vi "FocalChecker.vi"() -> ()   [LabVIEW 2016]
panel:
  out "Spectrum mean normalized 5":dbl[](graph)
  in  "File Path 5":path
  out "Spectrum mean normalized 4":dbl[](graph)
  in  "File Path 4":path
  out "Spectrum mean normalized 3":dbl[](graph)
  in  "File Path 3":path
  out "Spectrum mean normalized 2":dbl[](graph)
  in  "File Path 2":path
  in  "length Y":i32
  in  "index Y":i32
  in  "length X":i32
  in  "index X":i32
  in  "Multiplicator":dbl
  out "Spectrum mean normalized":dbl[](graph)
  in  "File Path":path
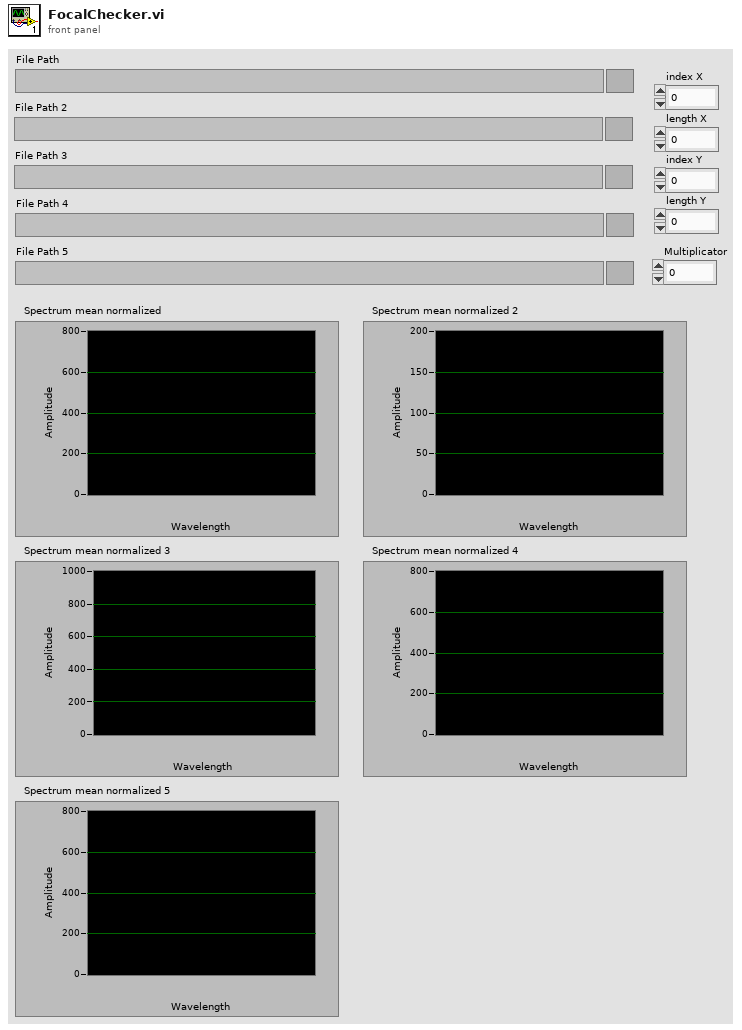
[diagram p1: front panel]
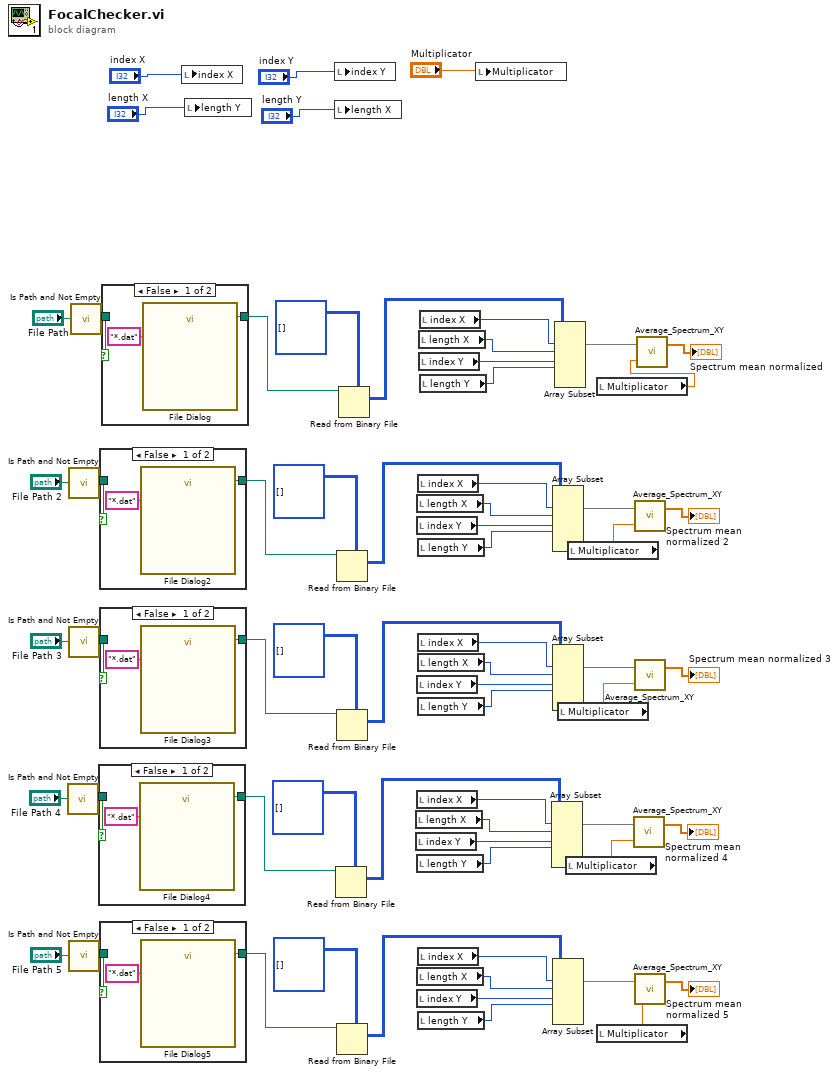
[diagram p0: block diagram]
diagram:
  n1 = call <vilib>:"Is Path and Not Empty.vi"("path"="File Path 4") -> ("Is Path and Not Empty?"=w26:bool)  [unwired: 4 in]
  n2 = call <vilib>:"Is Path and Not Empty.vi"("path"="File Path 2") -> ("Is Path and Not Empty?"=w48:bool)  [unwired: 4 in]
  n3 = call <vilib>:"Is Path and Not Empty.vi"("path"="File Path 3") -> ("Is Path and Not Empty?"=w37:bool)  [unwired: 4 in]
  n4 = call <vilib>:"Is Path and Not Empty.vi"("path"="File Path 5") -> ("Is Path and Not Empty?"=w15:bool)  [unwired: 4 in]
  n5 = call <vilib>:"Is Path and Not Empty.vi"("path"="File Path") -> ("Is Path and Not Empty?"=w64:bool)  [unwired: 4 in]
  n6 = case shown="False" w26 {
    tunnel: [w67 w68] -> w27
    tunnel: "File Path 4" -> [_ w68]
    frame False {
      n7 = call "File Dialog4"("pattern (all files)"="*.dat") -> ("selected path"=w67:path)  [unwired: 11 in, 3 out]
    }
    frame True {
    }
  }
  n8 = case shown="False" w48 {
    tunnel: [w70 w71] -> w49
    tunnel: "File Path 2" -> [_ w71]
    frame False {
      n9 = call "File Dialog2"("pattern (all files)"="*.dat") -> ("selected path"=w70:path)  [unwired: 11 in, 3 out]
    }
    frame True {
    }
  }
  n10 = case shown="False" w37 {
    tunnel: [w73 w74] -> w38
    tunnel: "File Path 3" -> [_ w74]
    frame False {
      n11 = call "File Dialog3"("pattern (all files)"="*.dat") -> ("selected path"=w73:path)  [unwired: 11 in, 3 out]
    }
    frame True {
    }
  }
  n12 = case shown="False" w15 {
    tunnel: [w76 w77] -> w16
    tunnel: "File Path 5" -> [_ w77]
    frame False {
      n13 = call "File Dialog5"("pattern (all files)"="*.dat") -> ("selected path"=w76:path)  [unwired: 11 in, 3 out]
    }
    frame True {
    }
  }
  n14 = case shown="False" w64 {
    tunnel: [w79 w80] -> w65
    tunnel: "File Path" -> [_ w80]
    frame False {
      n15 = call "File Dialog"("pattern (all files)"="*.dat") -> ("selected path"=w79:path)  [unwired: 11 in, 3 out]
    }
    frame True {
    }
  }
  n16 = local write "index X"("index X") -> ()
  n17 = local write "length Y"("length X") -> ()
  n18 = local write "index Y"("index Y") -> ()
  n19 = local write "length X"("length Y") -> ()
  n20 = Read from Binary File(5:u32[][][] [], 11:w27) -> (2:w21:u32[][][])  [unwired: 4 in, 3 out]
  n21 = Read from Binary File(5:u32[][][] [], 11:w49) -> (2:w43:u32[][][])  [unwired: 4 in, 3 out]
  n22 = Read from Binary File(5:u32[][][] [], 11:w38) -> (2:w32:u32[][][])  [unwired: 4 in, 3 out]
  n23 = Read from Binary File(5:u32[][][] [], 11:w16) -> (2:w10:u32[][][])  [unwired: 4 in, 3 out]
  n24 = Read from Binary File(5:u32[][][] [], 11:w65) -> (2:w59:u32[][][])  [unwired: 4 in, 3 out]
  n25 = local read "length X"() -> (w19:i32)
  n26 = local read "index Y"() -> (w18:i32)
  n27 = local read "length X"() -> (w41:i32)
  n28 = local read "index Y"() -> (w40:i32)
  n29 = local read "index Y"() -> (w29:i32)
  n30 = local read "index X"() -> (w20:i32)
  n31 = local read "length Y"() -> (w17:i32)
  n32 = local read "length X"() -> (w8:i32)
  n33 = local read "index Y"() -> (w7:i32)
  n34 = local read "index X"() -> (w42:i32)
  n35 = local read "length Y"() -> (w39:i32)
  n36 = local read "index X"() -> (w31:i32)
  n37 = local read "length X"() -> (w30:i32)
  n38 = local read "length Y"() -> (w28:i32)
  n39 = local read "index X"() -> (w9:i32)
  n40 = local read "length Y"() -> (w6:i32)
  n41 = local read "length X"() -> (w52:i32)
  n42 = local read "index Y"() -> (w51:i32)
  n43 = local read "index X"() -> (w53:i32)
  n44 = local read "length Y"() -> (w50:i32)
  n45 = local write "Multiplicator"("Multiplicator") -> ()
  n46 = Array Subset(array=w21, index (dim 0)=w20, length (dim 0)=w19, index (dim 1)=w18, length (dim 1)=w17) -> (w24:u32[][][])  [unwired: 2 in]
  n47 = Array Subset(array=w43, index (dim 0)=w42, length (dim 0)=w41, index (dim 1)=w40, length (dim 1)=w39) -> (w46:u32[][][])  [unwired: 2 in]
  n48 = Array Subset(array=w32, index (dim 0)=w31, length (dim 0)=w30, index (dim 1)=w29, length (dim 1)=w28) -> (w35:u32[][][])  [unwired: 2 in]
  n49 = Array Subset(array=w10, index (dim 0)=w9, length (dim 0)=w8, index (dim 1)=w7, length (dim 1)=w6) -> (w13:u32[][][])  [unwired: 2 in]
  n50 = Array Subset(array=w59, index (dim 0)=w53, length (dim 0)=w52, index (dim 1)=w51, length (dim 1)=w50) -> (w62:u32[][][])  [unwired: 2 in]
  n51 = local read "Multiplicator"() -> (w2:dbl)
  n52 = local read "Multiplicator"() -> (w3:dbl)
  n53 = local read "Multiplicator"() -> (w1:dbl)
  n54 = local read "Multiplicator"() -> (w5:dbl)
  n55 = local read "Multiplicator"() -> (w4:dbl)
  n56 = call "Average_Spectrum_XY.vi"("Multiplyer"=w3, "Array IN 3D"=w24) -> ("Array Out 1D"=→"Spectrum mean normalized 4":dbl[])  [unwired: 1 out]
  n57 = call "Average_Spectrum_XY.vi"("Multiplyer"=w1, "Array IN 3D"=w46) -> ("Array Out 1D"=→"Spectrum mean normalized 2":dbl[])  [unwired: 1 out]
  n58 = call "Average_Spectrum_XY.vi"("Multiplyer"=w2, "Array IN 3D"=w35) -> ("Array Out 1D"=→"Spectrum mean normalized 3":dbl[])  [unwired: 1 out]
  n59 = call "Average_Spectrum_XY.vi"("Multiplyer"=w4, "Array IN 3D"=w13) -> ("Array Out 1D"=→"Spectrum mean normalized 5":dbl[])  [unwired: 1 out]
  n60 = call "Average_Spectrum_XY.vi"("Multiplyer"=w5, "Array IN 3D"=w62) -> ("Array Out 1D"=→"Spectrum mean normalized":dbl[])  [unwired: 1 out]
